vi "test 2- NonCSMCallsSysLevelMode_UseAPI.vi"(8 "error in (no error)":errorcluster, 11 "TestCase in":refnum<class "testcase-SyncMessage.lvclass">) -> (0 "error out":errorcluster, 3 "TestCase out":refnum<class "testcase-SyncMessage.lvclass">)   [LabVIEW 2017, in "testcase-SyncMessage.lvclass"]
uses:
  testcase-SyncMessage.lvclass
  _support/SyncMessage_CSM_Callee.vi
  <vilib>/addons/_JKI Toolkits/VI Tester/TestCase.llb/TestCase.lvclass
  src/user.lib/_NEVSTOP/Communicable State Machine(CSM)/Communicable State Machine.lvlib
  C:/Program Files (x86)/National Instruments/LabVIEW 2017/vi.lib/addons/_JKI Toolkits/VI Tester/TestCase.llb/TestCase.lvclass
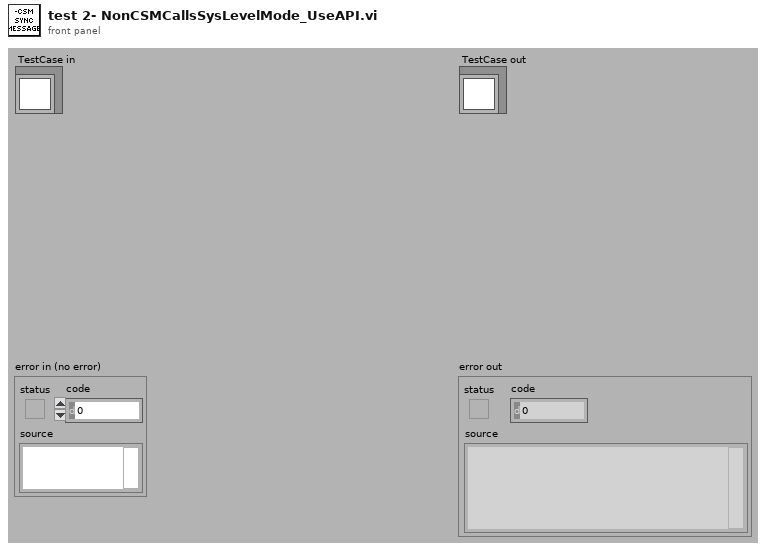
[diagram p1: front panel]
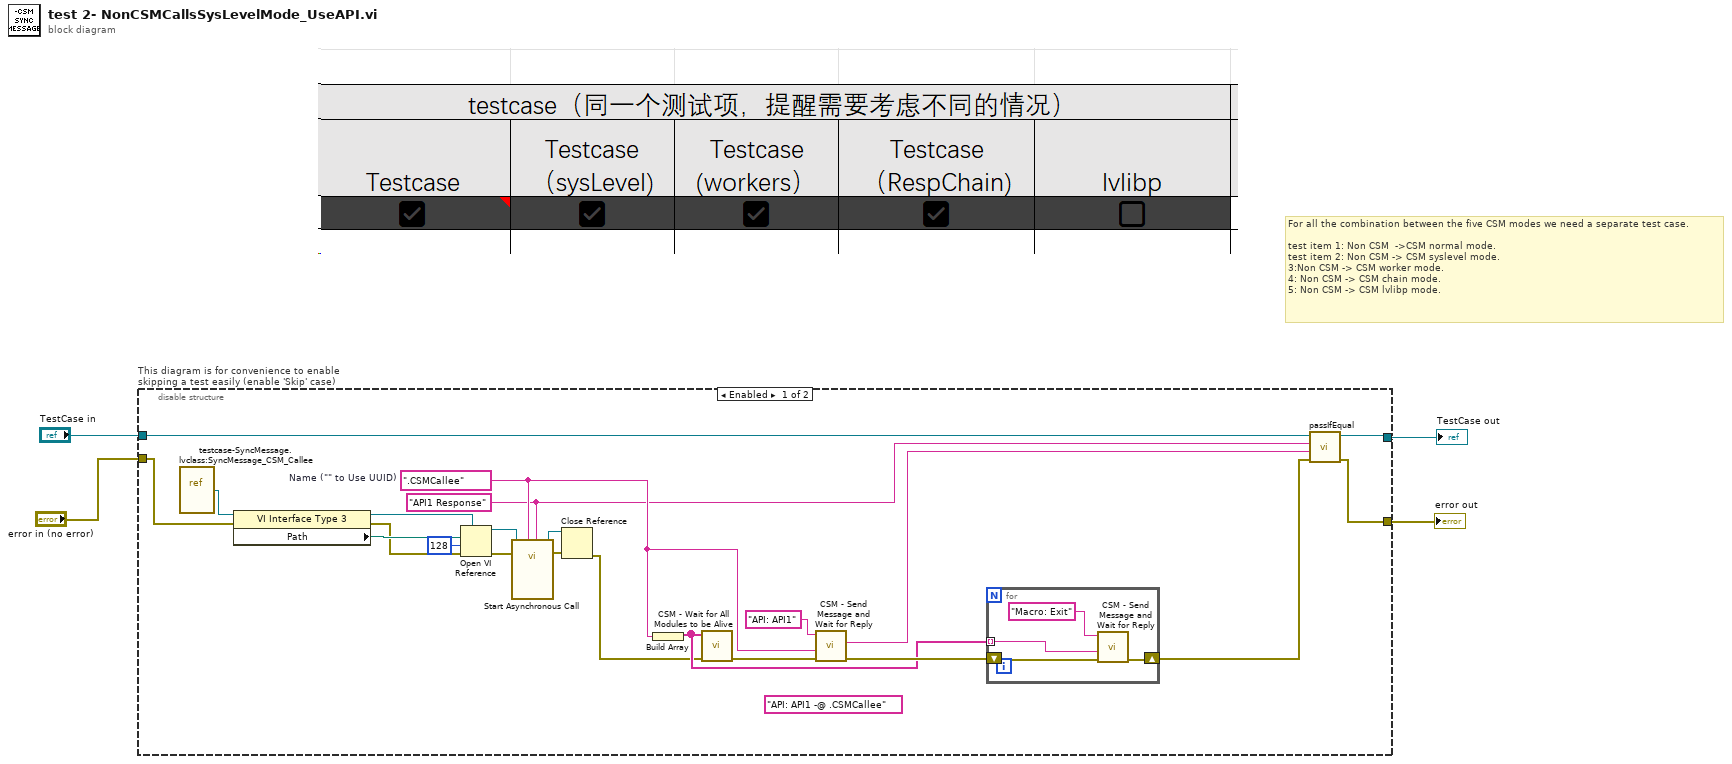
[diagram p0: block diagram]
diagram:
  # "For all the combination between the five CSM modes we need a separate test case.\n\ntest item 1: Non CSM  ->CSM normal mode.\ntest item 2: Non CSM -> CSM syslevel mode.\n3:Non CSM -> CSM worker mode.\n4: Non CSM -> CSM chain mode.\n5: Non CSM -> CSM lvlibp mode."
  n1 = disable-structure "This diagram is for convenience to enable skipping a test easily (enable 'Skip' case)" shown="Enabled" {
    disable-tunnel: "TestCase in" -> [w26 w34]
    disable-tunnel: [w25 w32] -> w2
    disable-tunnel: [w24 w33] -> w1
    disable-tunnel: "error in (no error)" -> [w8 w31]
    frame Enabled {
      w5 = "API1 Response" ("API response in")
      w6 = ".CSMCallee"  # Name ("" to Use UUID)
      (unwired) "API: API1 -@ .CSMCallee" ("Intermodule Message in")
      n2 = vi-ref "testcase-SyncMessage.lvclass:SyncMessage_CSM_Callee.vi"() -> (w16:refnum<vi>)
      n3 = property class="VI Interface Type 3"(reference=w16, error in=w8) -> (reference out=w12:refnum<vi>, error out=w14:errorcluster, "Path"=w15:path)
      n4 = Open VI Reference(type specifier VI Refnum (for type only)=w12, vi path=w15, options=128, error in (no error)=w14) -> (vi reference=w13:refnum<vi>, error out=w17:errorcluster)  [unwired: 2 in]
      n5 = call-by-ref "Start Asynchronous Call"(reference=w13, error in=w17, "API response in"=w5, "Name (\"\" to Use UUID)"=w6) -> (reference out=w10:refnum<vi>, error out=w11:errorcluster)  [unwired: 10 in]
      n6 = Close Reference(reference=w10, error in (no error)=w11) -> (error out=w7:errorcluster)
      n7 = Build Array(w6) -> (w18:string[])
      n8 = call "CSM - Wait for All Modules to be Alive.vi"("Error In"=w7, "CSM Names"=w18) -> ("error out"=w22:errorcluster)  [unwired: 7 in, 2 out]
      n9 = call "CSM - Send Message and Wait for Reply.vi"("Error In (No Error)"=w22, "Target Module"=w6, "State"="API: API1") -> ("error out"=w19:errorcluster, "Response"=w20:string)  [unwired: 6 in, 1 out]
      n10 = for {
        shift-right: [w29] -> w23
        shift-left: w19 -> [w30]
        tunnel: w18 -> [w27] mode=indexing
        n11 = call "CSM - Send Message and Wait for Reply.vi"("Error In (No Error)"=w30, "Target Module"=w27, "State"="Macro: Exit") -> ("error out"=w29:errorcluster)  [unwired: 6 in, 2 out]
      }
      n12 = call-dynamic "passIfEqual.vi"("error in (no error)"=w23, "y"=w20, "x"=w5, "TestCase in"=w26) -> ("error out"=w24:errorcluster, "TestCase out"=w25:refnum<class "testcase-SyncMessage.lvclass">)  [unwired: 6 in]
    }
    frame Disabled {
      # "skip test result while test is under development"
      n13 = call <vilib>:"skip.vi"("error in (no error)"=w31, "TestCase in"=w34) -> ("error out"=w33:errorcluster, "TestCase out"=w32:refnum<class "testcase-SyncMessage.lvclass">)  [unwired: 8 in]
    }
  }
  "error out" <- w1
  "TestCase out" <- w2
